vi "Obtain and Save.vi"(8 "error in (no error)":errorcluster, 11 "LogsAbstract in":refnum<class "LogsAbstract.lvclass">) -> (0 "error out":errorcluster, 3 "LogsAbstract out":refnum<class "LogsAbstract.lvclass">)   [LabVIEW 2019, in "LogsAbstract.lvlib" / "LogsAbstract.lvclass"]
uses:
  LogsAbstract.lvclass
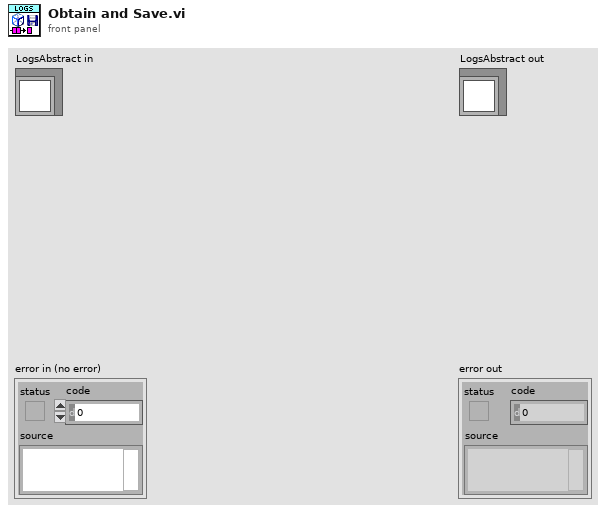
[diagram p1: front panel]
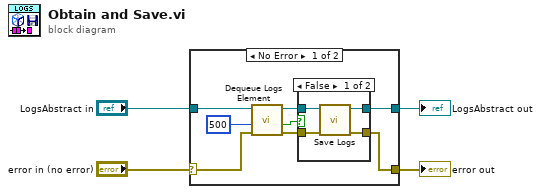
[diagram p0: block diagram]
diagram:
  n1 = case shown="No Error" "error in (no error)" {
    selector: "error in (no error)" -> [w9 w20]
    tunnel: [w7 w20] -> w3
    tunnel: [w10 w19] -> w1
    tunnel: "LogsAbstract in" -> [w12 w19]
    frame No Error {
      n2 = call-dynamic "Dequeue Logs Element.vi"("Error In"=w9, "Timeout"=500, "EventLog in"=w12) -> ("Error Out"=w8:errorcluster, "Timed out?"=w6:bool, "EventLog out"=w11:refnum<class "LogsAbstract.lvclass">)  [unwired: 6 in]
      n3 = case shown="False" w6 {
        tunnel: w11 -> [w16 w18]
        tunnel: [w15 w18] -> w10
        tunnel: w8 -> [w14 w17]
        tunnel: [w13 w17] -> w7
        frame False {
          n4 = call-dynamic "Save Logs.vi"("Error In"=w14, "EventLog in"=w16) -> ("Error Out"=w13:errorcluster, "EventLog out"=w15:refnum<class "LogsAbstract.lvclass">)  [unwired: 8 in]
        }
        frame True {
        }
      }
    }
    frame Error {
    }
  }
  "error out" <- w3
  "LogsAbstract out" <- w1
